vi "Oil Pump Speed.vi"(10 "Controller Toggle P 2":bool, 11 "Compressor Input":T2={"Compressor Speed Adjust"=100.0, "Accept Autotune Water Pump"=FALSE, "Fine slide in P"=refnum, "file for water pump"=path "", "autotune? water pump"=FALSE, "PID gains in water pump"={"proportional gain (Kc)"=0.0, "integral time (Ti, min)"=0.0, "derivative time (Td, min)"=0.0}} {"Compressor Speed Adjust" min=0.0 max=100.0 step=1.0 scale=0.0..100.0}) -> (3 "output cluster":T1)   [LabVIEW 2017]
panel:
  out "output to valve":dbl
  in  "Reinitialize Controller":bool
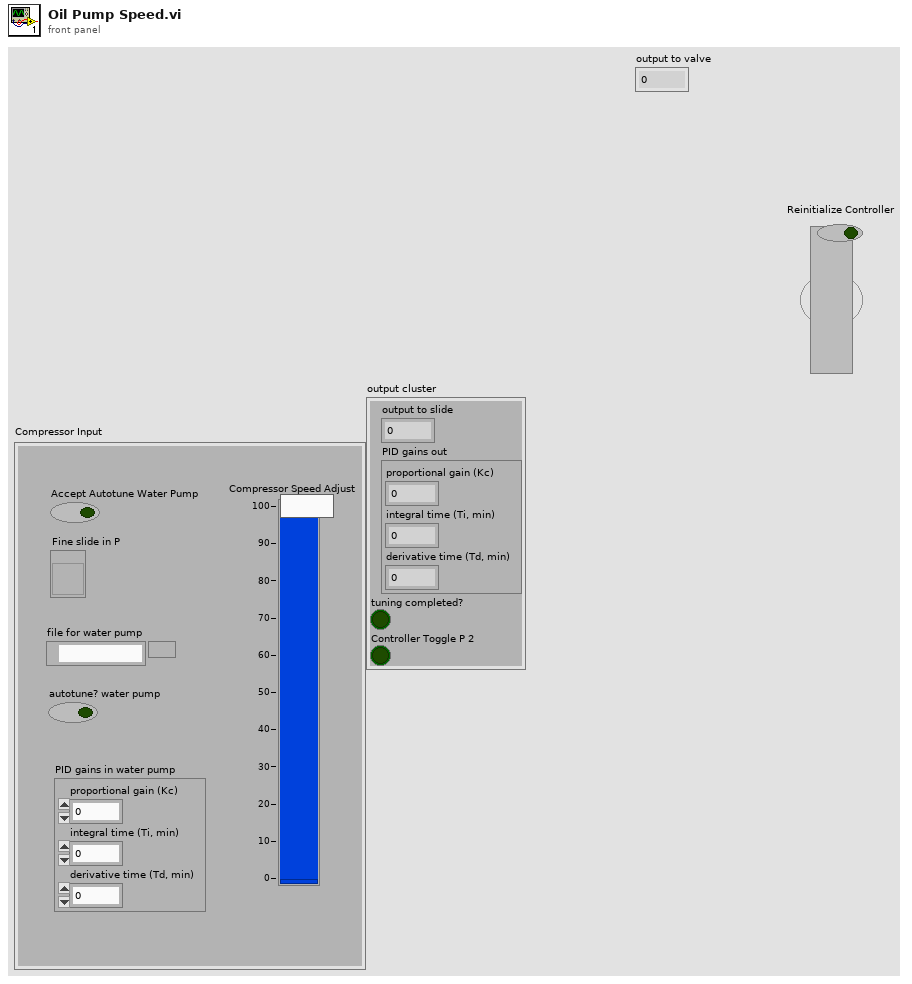
[diagram p1: front panel]
types:
  T1 = cluster{"output to slide":dbl, "PID gains out":cluster{"proportional gain (Kc)":dbl, "integral time (Ti, min)":dbl, "derivative time (Td, min)":dbl}, "tuning completed?":bool, "Controller Toggle P 2":bool}
  T2 = cluster{"Compressor Speed Adjust":dbl, "Accept Autotune Water Pump":bool, "Fine slide in P":refnum<vi>, "file for water pump":path, "autotune? water pump":bool, "PID gains in water pump":cluster{"proportional gain (Kc)":dbl, "integral time (Ti, min)":dbl, "derivative time (Td, min)":dbl}}
  T3 = cluster{"proportional gain (Kc)":dbl, "integral time (Ti, min)":dbl, "derivative time (Td, min)":dbl}
  T4 = enum8{"Enabled", "Disabled", "Disabled and Grayed Out"}
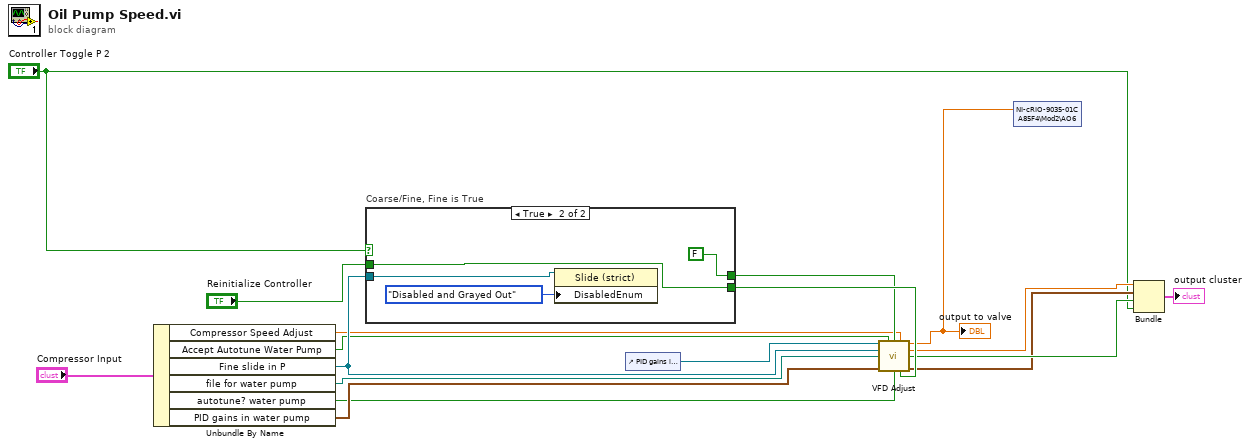
[diagram p0: block diagram]
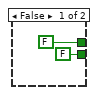
[diagram p2: hidden frame]
diagram:
  n1 = Unbundle By Name("Compressor Input") -> ("Compressor Speed Adjust"=w7:dbl, "Accept Autotune Water Pump"=w9:bool, "Fine slide in P"=w13:refnum<vi>, "file for water pump"=w14:path, "autotune? water pump"=w10:bool, "PID gains in water pump"=w15:T3)
  n2 = case "Coarse/Fine, Fine is True" shown="True" "Controller Toggle P 2" {
    tunnel: "Reinitialize Controller" -> [_ w20]
    tunnel: [FALSE w20] -> w11
    tunnel: [FALSE FALSE] -> w8
    tunnel: w13 -> [_ w21]
    frame False {
    }
    frame True {
      n3 = property on="Property Node" class="Slide (strict)"(reference=w21, "DisabledEnum"=T4."Disabled and Grayed Out" ("Disabled")) -> ()  [unwired: 1 in, 2 out]
    }
  }
  n4 = control-ref of="PID gains in water pump"() -> (w12:refnum<vi>)
  n5 = call "VFD Adjust.vi"("PID Gains Cluster Ref"=w12, "Accept Autotune"=w9, "Controller Toggle (Manual Mode)"=w8, "Valve Manual Adjust"=w7, "Slide Refnum in"=w13, "file (use dialog)"=w14, "PID gains"=w15, "autotune? (F)"=w10, "Reinitialize Controller"=w11) -> ("output to valve"=w1:dbl, "output to slide"=w6:dbl, "tuning completed?"=w5:bool, "PID gains out"=w4:T3)  [unwired: 2 in, 1 out]
  "output to valve" <- w1
  n6 = shared-variable "NI-cRIO-9035-01CA85F4\\Mod2\\AO6"(w1) -> ()  [unwired: 1 in, 1 out]
  n7 = Bundle("output to slide"=w6, "PID gains out"=w4, "tuning completed?"=w5, "Controller Toggle P 2"="Controller Toggle P 2") -> (→"output cluster":T1)  [unwired: 1 in]
